vi "tip_cal_error.vi"(9 "X":dbl[](array[numeric]), 11 "Calibration point pose":dbl[][][](array[numeric])) -> (0 "Residuals":dbl[](array[numeric]), 2 "f(X)":dbl)   [LabVIEW 2013]
uses:
  <vilib>/Analysis/baseanly.llb/A x Vector.vi
  <vilib>/Analysis/NI_AALBase.lvlib
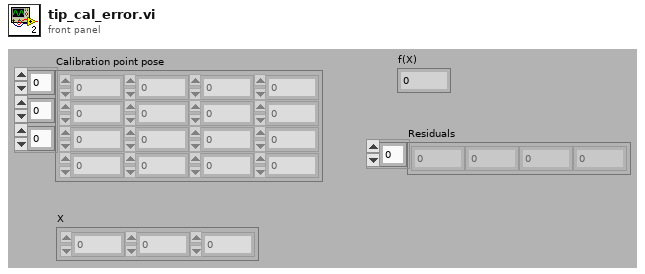
[diagram p1: front panel]
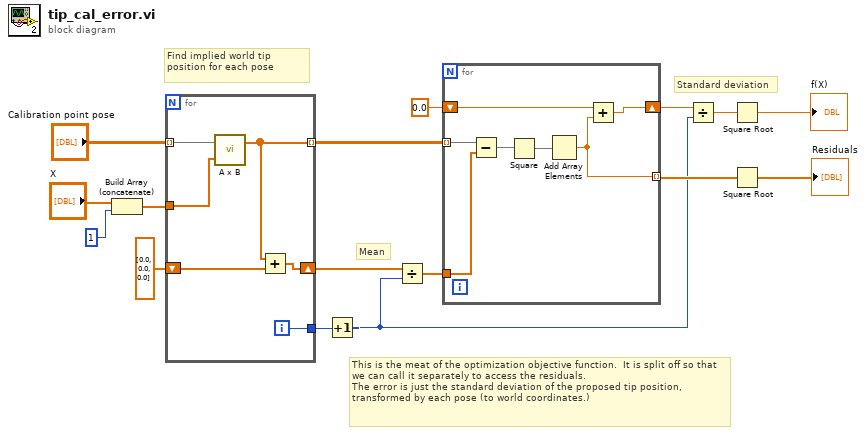
[diagram p0: block diagram]
diagram:
  # "This is the meat of the optimization objective function.  It is split off so that we can call it separately to access the residuals.\nThe error is just the standard deviation of the proposed tip position, transformed by each pose (to world coordinates.)"
  # "Standard deviation"
  # "Mean"
  # "Find implied world tip position for each pose"
  n1 = Build Array (concatenate)("X", 1 ("Numeric")) -> (w15:dbl[])
  n2 = for {
    tunnel: "Calibration point pose" -> [w22] mode=indexing
    tunnel: w15 -> [w21]
    tunnel: [w18] -> w8 mode=indexing
    tunnel: [w20] -> w2
    shift-right: [w17] -> w7
    shift-left: dbl[] [0.0, 0.0, 0.0] ("A x Vector") -> [w19]
    i -> [w20]
    n3 = call-poly <vilib>:"A x B.vi"("Vector"=w21, "A"=w22) -> ("A x Vector"=w18:dbl[])  [unwired: 1 out]
    n4 = Add(x=w18, y=w19) -> (x+y=w17:dbl[])
  }
  n5 = Increment(x=w2) -> (x+1=w1:i32)
  n6 = Divide(x=w7, y=w1) -> (x/y=w9:dbl[])
  n7 = for {
    tunnel: w8 -> [w29] mode=indexing
    tunnel: w9 -> [w28]
    shift-right: [w26] -> w11
    shift-left: 0.0 ("f(X)") -> [w25]
    tunnel: [w23] -> w4 mode=indexing
    n8 = Subtract(x=w29, y=w28) -> (x-y=w27:dbl[])
    n9 = Square(x=w27) -> (x^2=w24:dbl[])
    n10 = Add Array Elements(numeric array=w24) -> (sum=w23:dbl)
    n11 = Add(x=w25, y=w23) -> (x+y=w26:dbl)
  }
  n12 = Divide(x=w11, y=w1) -> (x/y=w12:dbl)
  n13 = Square Root(x=w12) -> (sqrt(x)=→"f(X)":dbl)
  n14 = Square Root(x=w4) -> (sqrt(x)=→"Residuals":dbl[])
